vi "RT Error Handler - Host Messaging Loop.vi"(1 "Error In":errorcluster, 2 "Message Queue":refnum<queue>) -> ()   [LabVIEW 2017]
uses:
  Support/Message Queue/Message Cluster.ctl
  Support/Message Queue/Message Queue.lvlib
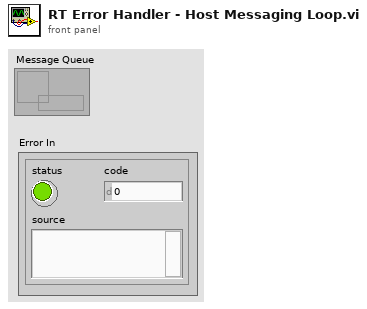
[diagram p1: front panel]
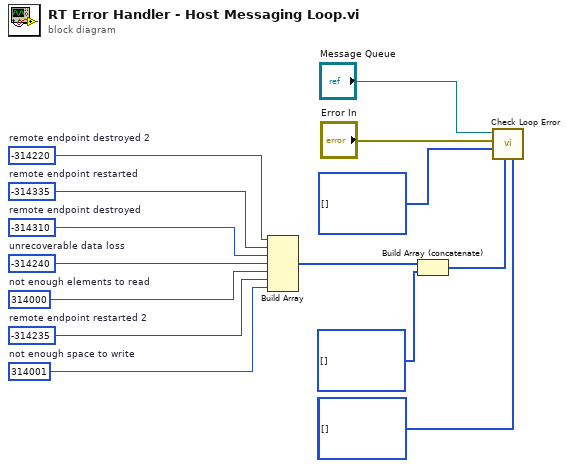
[diagram p0: block diagram]
diagram:
  w4 = -314220  # remote endpoint destroyed 2
  w5 = 314001  # not enough space to write
  w7 = 314000  # not enough elements to read
  w6 = -314235  # remote endpoint restarted 2
  w8 = -314240  # unrecoverable data loss
  w9 = -314310  # remote endpoint destroyed
  w10 = -314335  # remote endpoint restarted
  (unwired) i32[] [] ("Critical Errors")
  n1 = Build Array(w4, w10, w9, w8, w7, w6, w5) -> (w2:i32[])
  n2 = Build Array (concatenate)(w2, i32[] [] ("Critical Errors")) -> (w3:i32[])
  n3 = call "Check Loop Error.vi"("Ignore Errors"=i32[] [-314004] ("Critical Errors"), "Log-Only Errors"=w3, "Critical Errors"=i32[] [], "error to process"="Error In", "Message Queue"="Message Queue") -> ()  [unwired: 5 in, 2 out]
